vi "Comm Connect.vi"(8 "error in (no error)":errorcluster, 11 "niDTS Comm EXE in":refnum<class "niDTS Comm EXE.lvclass">) -> (0 "error out":errorcluster, 3 "niDTS Comm EXE out":refnum<class "niDTS Comm EXE.lvclass">)   [LabVIEW 2015, in "niDTS CommLib.lvlib" / "niDTS Comm EXE.lvclass"]
uses:
  niDTS Comm EXE.lvclass
  Framework/Logger/Includes/niDTS Logger INC Log Element Type.ctl
  Framework/Logger/Objects/BASE_class/niDTS Logger.lvclass
  Framework/niDTS Framework.lvlib
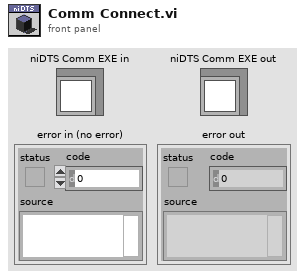
[diagram p1: front panel]
types:
  T1 = typedef "niDTS Framework.lvlib/niDTS Logger INC Handle.ctl" = refnum<data-value>
  T2 = typedef "niDTS Framework.lvlib/niDTS Logger INC Log Element Type.ctl" = enum16{"Error", "Warning", "Information", "Debugging"}
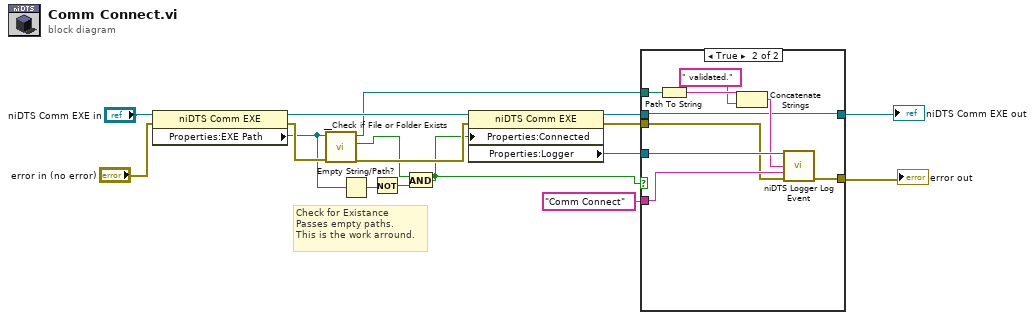
[diagram p0: block diagram]
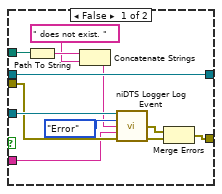
[diagram p2: hidden frame]
diagram:
  # "Check for Existance\nPasses empty paths.\nThis is the work arround."
  n1 = property class="niDTS Comm EXE"(reference="niDTS Comm EXE in", error in="error in (no error)") -> (reference out=w16:refnum<class "niDTS Comm EXE.lvclass">, error out=w13:errorcluster, "Properties:EXE Path"=w4:path)
  n2 = call "__Check if File or Folder Exists.vi"("error in (no error)"=w13, "path"=w4) -> ("error out"=w12:errorcluster, "file or folder exists?"=w2:bool, "dup path"=w10:path)  [unwired: 7 in]
  n3 = Empty String/Path?(string/path=w4) -> (empty?=w5:bool)
  n4 = Not(x=w5) -> (.not. x?=w3:bool)
  n5 = And(x=w2, y=w3) -> (x .and. y?=w1:bool)
  n6 = property class="niDTS Comm EXE"(reference=w16, error in=w12, "Properties:Connected"=w1) -> (reference out=w15:refnum<class "niDTS Comm EXE.lvclass">, error out=w9:errorcluster, "Properties:Logger"=w11:T1)
  n7 = case shown="True" w1 {
    tunnel: w15 -> [w24 w32]
    tunnel: w11 -> [w28 w38]
    tunnel: w10 -> [w27 w36]
    tunnel: [w24 w32] -> w7
    tunnel: w9 -> [w23 w30]
    tunnel: [w22 w31] -> w8
    tunnel: "Comm Connect" ("Source/Location") -> [w21 w37]
    frame False {
      n8 = Path To String(path=w27) -> (string=w26:string)
      n9 = Concatenate Strings(w26, " does not exist. " ("string")) -> (w20:string)
      n10 = call "niDTS Logger Log Event.vi"("Logger Handle"=w28, "Type"=niDTS_Logger_INC_Log_Element_Type."Error", "Description/Data"=w20, "Source/Location"=w21, "error in (no error)"=w23) -> ("Source Data Error"=w18:errorcluster, "error out"=w19:errorcluster)  [unwired: 8 in, 1 out]
      n11 = Merge Errors(w18, w19) -> (w22:errorcluster)
    }
    frame True {
      n12 = Path To String(path=w36) -> (string=w35:string)
      n13 = Concatenate Strings(w35, " validated." ("string")) -> (w33:string)
      n14 = call "niDTS Logger Log Event.vi"("Logger Handle"=w38, "Description/Data"=w33, "Source/Location"=w37, "error in (no error)"=w30) -> ("error out"=w31:errorcluster)  [unwired: 9 in, 2 out]
    }
  }
  "error out" <- w8
  "niDTS Comm EXE out" <- w7
